vi "Create MQTT Client.vi"(8 "error in":errorcluster, 9 "Remote Port":u16, 10 "IP Address":string, 11 "Module ID":i32) -> (0 "error out":errorcluster, 1 "Client out":refnum<class "Client.lvclass">, 2 "MQTT Public Events":T1, 3 "Client Public Events":T2, 4 "Error connecting?":bool)   [LabVIEW 2016, in "MQTT_Client.lvlib"]
uses:
  MQTT_Client.lvlib
  <vilib>/LabVIEW Open Source Project/MQTT Client/Client class/Client.lvclass
  <vilib>/LabVIEW Open Source Project/MQTT Control Packets/Control Packets/CONNECT/ConnectFlags -- cluster.ctl
  <vilib>/LabVIEW Open Source Project/MQTT Control Packets/Control Packets/CONNECT/CONNECT.lvclass
  <vilib>/LabVIEW Open Source Project/MQTT Connection/MQTT_Base/Base Class/MQTT_Base.lvclass
  <vilib>/LabVIEW Open Source Project/MQTT TCP Connection/MQTT_TCP/Connection/TCPConnection.lvclass
  C:/Program Files (x86)/National Instruments/LabVIEW 2020/vi.lib/LabVIEW Open Source Project/MQTT Connection/MQTT_Base/Base Class/MQTT_Base.lvclass
  <vilib>/LabVIEW Open Source Project/OpenSerializer JKI JSON/Serializer.JSON.lvclass
  C:/Program Files (x86)/National Instruments/LabVIEW 2020/vi.lib/LabVIEW Open Source Project/MQTT Connection/MQTT_Connection/Connection/Connection.lvclass
  C:/Program Files (x86)/National Instruments/LabVIEW 2020/vi.lib/LabVIEW Open Source Project/Connection/Connection/Connection.lvclass
  C:/Program Files (x86)/National Instruments/LabVIEW 2020/vi.lib/LabVIEW Open Source Project/OpenSerializer/Serializer/Serializer.lvclass
  <vilib>/LabVIEW Open Source Project/MQTT Control Packets/Control Packets/CONNACK/Connect Return Code -- enum.ctl
  <vilib>/LabVIEW Open Source Project/MQTT Control Packets/Control Packets/CONNACK/CONNACK.lvclass
  <vilib>/LabVIEW Open Source Project/MQTT Control Packets/Control Packets/PUBLISH/PUBLISH.lvclass
  <vilib>/LabVIEW Open Source Project/MQTT Client/Client class/Public Events -- cluster.ctl
  <vilib>/LabVIEW Open Source Project/MQTT Connection/MQTT_Base/Base Class/Public Events -- cluster.ctl
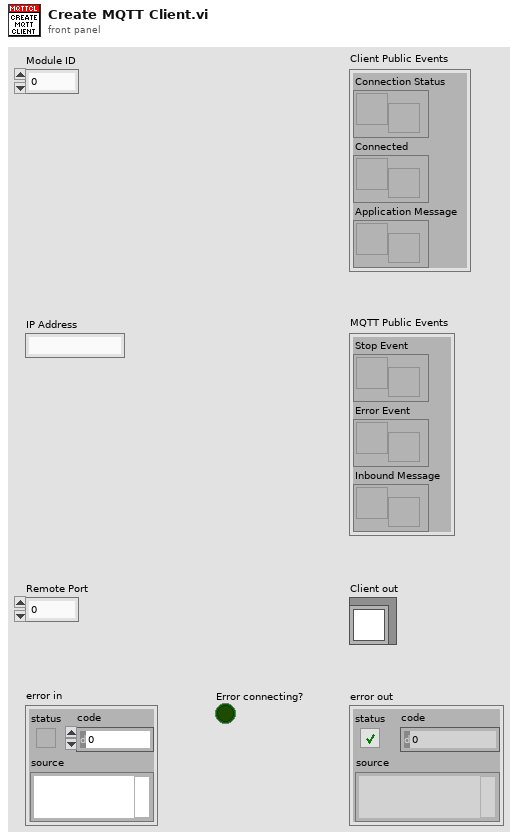
[diagram p1: front panel]
types:
  T1 = typedef "MQTT Base.lvlib/MQTT_Base.lvclass/Public Events -- cluster.ctl" = cluster{"Stop Event":refnum<user-event>, "Error Event":refnum<user-event>, "Inbound Message":refnum<user-event>}
  T2 = typedef "MQTT Client.lvlib/Client.lvclass/Public Events -- cluster.ctl" = cluster{"Connection Status":refnum<user-event>, "Connected":refnum<user-event>, "Application Message":refnum<user-event>}
  T3 = typedef "MQTT_Control_Packets.lvlib/CONNECT.lvclass/ConnectFlags -- cluster.ctl" = cluster{"Reserved":bool, "Clean Session":bool, "Will Flag":bool, "Will QoS 1":bool, "Will QoS 2":bool, "Will Retain":bool, "Password Flag":bool, "User Name Flag":bool}
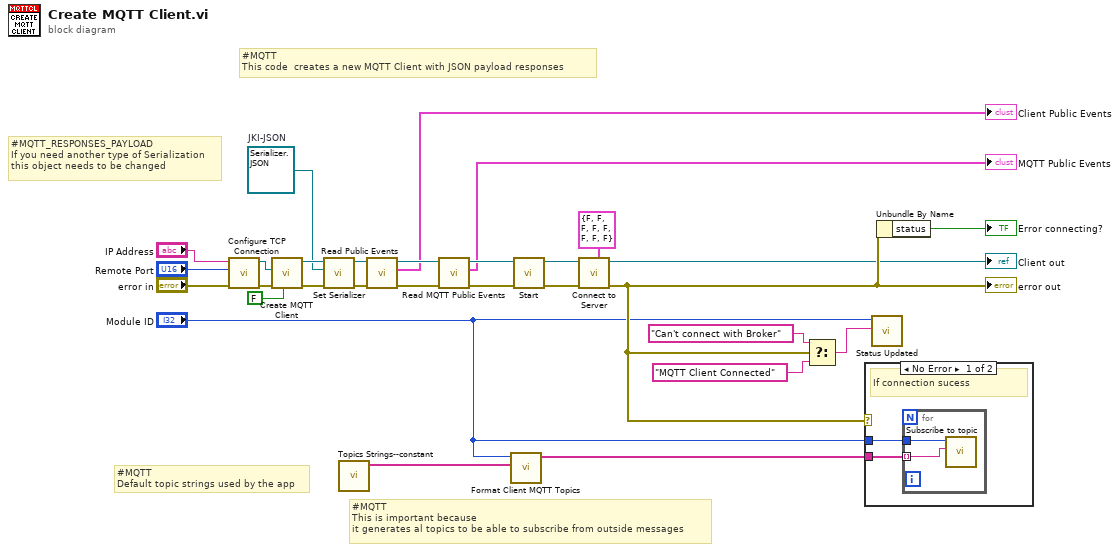
[diagram p0: block diagram]
diagram:
  w3 = refnum<class "Serializer.JSON.lvclass"> refnum  # JKI-JSON
  # "#MQTT   \nDefault topic strings used by the app"
  # "#MQTT   \nThis is important because\nit generates al topics to be able to subscribe from outside messages"
  # "#MQTT_RESPONSES_PAYLOAD\nIf you need another type of Serialization\nthis object needs to be changed"
  # "#MQTT  \nThis code  creates a new MQTT Client with JSON payload responses"
  n1 = call <vilib>:"Configure TCP Connection.vi"("error in (no error)"="error in", "remote port (80)"="Remote Port", "address (localhost)"="IP Address") -> ("error out"=w26:errorcluster, "TCPConnection"=w10:refnum<class "TCPConnection.lvclass">)  [unwired: 7 in]
  n2 = call <vilib>:"Create MQTT Client.vi"("Enable Mutex ? (F)"=FALSE, "error in (no error)"=w26, "Connection Configuration"=w10) -> ("error out"=w28:errorcluster, "Client out"=w14:refnum<class "Client.lvclass">)  [unwired: 7 in]
  n3 = call <vilib>:"Set Serializer.vi"("error in (no error)"=w28, "Serializer (default: Flattened String)"=w3, "MQTT_Base"=w14) -> ("error out"=w29:errorcluster, "MQTT_Base out"=w15:refnum<class "Client.lvclass">)  [unwired: 7 in]
  n4 = call "Topics Strings--constant.vi"() -> ("Topics Strings"=w2:string[])  [unwired: 11 in]
  n5 = call <vilib>:"Read Public Events.vi"("error in (no error)"=w29, "Client in"=w15) -> ("error out"=w25:errorcluster, "Client Public Events"=→"Client Public Events":T2, "Client out"=w9:refnum<class "Client.lvclass">)  [unwired: 7 in]
  n6 = call <vilib>:"Read MQTT Public Events.vi"("error in (no error)"=w25, "MQTT_Base in"=w9) -> ("error out"=w23:errorcluster, "MQTT Public Events"=→"MQTT Public Events":T1, "MQTT_Base out"=w11:refnum<class "Client.lvclass">)  [unwired: 7 in]
  n7 = call "Format Client MQTT Topics.vi"("Topics Strings"=w2, "Module ID"="Module ID") -> ("Topics"=w5:string[])  [unwired: 9 in]
  n8 = call <vilib>:"Start.vi"("error in (no error)"=w23, "MQTT_Base in"=w11) -> ("error out"=w27:errorcluster, "MQTT_Base out"=w12:refnum<class "Client.lvclass">)  [unwired: 7 in, 1 out]
  n9 = call <vilib>:"Connect to Server.vi"("Connect Flags"=T3 {"Reserved"=FALSE, "Clean Session"=FALSE, "Will Flag"=FALSE, "Will QoS 1"=FALSE, "Will QoS 2"=FALSE, "Will Retain"=FALSE, "Password Flag"=FALSE, "User Name Flag"=FALSE}, "error in (no error)"=w27, "Client in"=w12) -> ("error out"=w22:errorcluster, "Client out"=→"Client out":refnum<class "Client.lvclass">)  [unwired: 5 in, 2 out]
  "error out" <- w22
  n10 = Select(t="Can't connect with Broker" ("Status"), s=w22, f="MQTT Client Connected" ("Status")) -> (s? t:f=w20:string)
  n11 = case shown="No Error" w22 {
    tunnel: "Module ID" -> [w31 _]
    tunnel: w5 -> [w30 _]
    frame No Error {
      # "If connection sucess"
      n12 = for {
        tunnel: w31 -> [w33]
        tunnel: w30 -> [w32] mode=indexing
        n13 = call "Subscribe to topic.vi"("Topic"=w32, "Module ID"=w33) -> ()  [unwired: 9 in, 1 out]
      }
    }
    frame Error {
    }
  }
  n14 = call "Status Updated.vi"("Status"=w20, "Module ID"="Module ID") -> ()  [unwired: 9 in, 1 out]
  n15 = Unbundle By Name(w22) -> ("status"=→"Error connecting?":bool)
